vi "SetCursorPos(ObjectName).vi"(8 "error in":errorcluster, 9 "Object Name":string, 10 "Front Panel Window:Open":bool=TRUE, 11 "VIpath":path) -> (0 "Error out":errorcluster, 3 "Sucess?":i32)   [LabVIEW 2013]
uses:
  <vilib>/Utility/miscctls.llb/LVPositionTypeDef.ctl
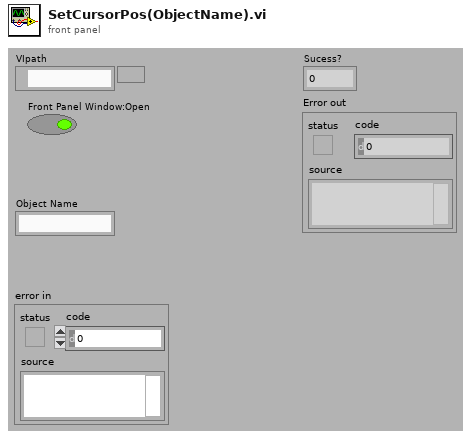
[diagram p1: front panel]
types:
  T1 = typedef "LVPositionTypeDef.ctl" = cluster{"Left":i32, "Top":i32}
  T2 = typedef "LVRectTypeDef.ctl" = cluster{"Left":i16, "Top":i16, "Right":i16, "Bottom":i16}
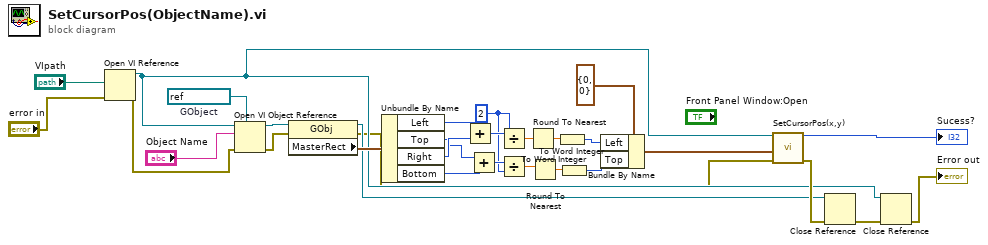
[diagram p0: block diagram]
diagram:
  w20 = i16 2 ("y")
  w30 = refnum<vi> refnum  # GObject
  n1 = Open VI Reference(vi path="VIpath", error in (no error)="error in") -> (vi reference=w2:refnum<vi>, error out=w9:errorcluster)  [unwired: 4 in]
  n2 = Open VI Object Reference(7:w30, 8:w9, 10:"Object Name", 11:w2) -> (0:w28:errorcluster, 3:w29:refnum<vi>)
  n3 = property class="GObj"(reference=w29, error in=w28) -> (reference out=w4:refnum<vi>, error out=w1:errorcluster, "MasterRect"=w27:T2)
  n4 = Unbundle By Name(w27) -> ("Left"=w26:i16, "Top"=w24:i16, "Right"=w25:i16, "Bottom"=w23:i16)
  n5 = Add(x=w26, y=w25) -> (x+y=w22:i16)
  n6 = Add(x=w24, y=w23) -> (x+y=w21:i16)
  n7 = Divide(x=w22, y=w20) -> (x/y=w19:dbl)
  n8 = Divide(x=w21, y=w20) -> (x/y=w18:dbl)
  n9 = Round To Nearest(number=w19) -> (nearest integer value=w17:dbl)
  n10 = Round To Nearest(number=w18) -> (nearest integer value=w16:dbl)
  n11 = To Word Integer(number=w17) -> (16bit integer=w15:i16)
  n12 = To Word Integer(number=w16) -> (16bit integer=w14:i16)
  n13 = Bundle By Name(cluster=T1 {"Left"=0, "Top"=0} ("x+y"), "Left"=w15, "Top"=w14) -> (w12:T1)
  n14 = call "SetCursorPos(x,y).vi"("vi reference"=w2, "(X,Y)"=w12, "Error in"=w1) -> ("Sucess?"=→"Sucess?":i32, "Error out"=w7:errorcluster)  [unwired: 11 in]
  n15 = Close Reference(reference=w4, error in (no error)=w7) -> (error out=w6:errorcluster)
  n16 = Close Reference(reference=w2, error in (no error)=w6) -> (error out=→"Error out":errorcluster)
